vi "Get Value (Boolean).vi"(8 "error in (no error)":errorcluster, 10 "key":string, 11 "JSON Object in":refnum<class "JSON Object.lvclass">) -> (0 "error out":errorcluster, 1 "found":bool, 2 "value":refnum<class "JSON Boolean.lvclass">)   [LabVIEW 2015, in "LVJSON.lvlib" / "JSON Object.lvclass"]
uses:
  JSON Object.lvclass
  JSON Boolean/JSON Boolean.lvclass
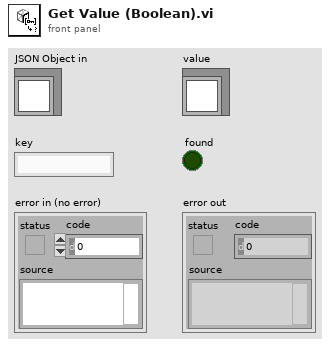
[diagram p1: front panel]
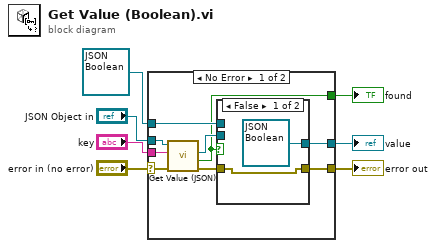
[diagram p0: block diagram]
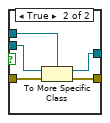
[diagram p2: hidden frame]
diagram:
  n1 = case shown="No Error" "error in (no error)" {
    selector: "error in (no error)" -> [w8 w25]
    tunnel: [w11 w25] -> w6
    tunnel: "JSON Object in" -> [w16 _]
    tunnel: "key" -> [w15 _]
    tunnel: [w13 w24] -> w2
    tunnel: refnum<class "JSON Boolean.lvclass"> refnum ("JSON Boolean.lvclass") -> [w10 w24]
    tunnel: [w9 _] -> w1
    frame No Error {
      n2 = call "Get Value (JSON).vi"("error in (no error)"=w8, "key"=w15, "JSON Object in"=w16) -> ("error out"=w12:errorcluster, "found"=w9:bool, "value"=w14:refnum<class "JSON Datatype.lvclass">)  [unwired: 6 in]
      n3 = case shown="False" w9 {
        tunnel: w14 -> [_ w23]
        tunnel: [refnum<class "JSON Boolean.lvclass"> refnum ("JSON Boolean.lvclass") w22] -> w13
        tunnel: w12 -> [w17 w21]
        tunnel: [w17 w20] -> w11
        tunnel: w10 -> [_ w19]
        frame False {
        }
        frame True {
          n4 = To More Specific Class(target class=w19, reference=w23, error in=w21) -> (specific class reference=w22:refnum<class "JSON Boolean.lvclass">, error out=w20:errorcluster)
        }
      }
    }
    frame Error {
    }
  }
  "error out" <- w6
  "value" <- w2
  "found" <- w1
